vi "extracted json single string.vi"(7 "Data Type and Default Value":string, 9 "error in (no error)":errorcluster, 10 "Offset":i32, 11 "JSON":string) -> (1 "error out":errorcluster, 3 "Data out":string)   [LabVIEW 2026]
doc: "Convert JSON to the LabVIEW Data Type entered.\n\nStrings or Arrays of strings marked with a leading \"<JSON>\" tag in their name (including inside clusters) are returnd as JSON. \n\nStrings or Arrays of strings marked with a leading \"<UTF8>\" tag in their name (including inside clusters) are returned encoded as UTF-8 (rather than the standard LabVIEW encoding)."
uses:
  <vilib>/JDP Science/JSONtext/JSONtext.lvlib
  <vilib>/Utility/Data Type/NI_Data Type.lvlib
  <vilib>/JDP Science/JDP Science Common Utilities/JDP Utility.lvlib
  <vilib>/Utility/Data Type/Type Definitions/Data Type.ctl
  <vilib>/JDP Science/JSONtext/support/Tag Type.ctl
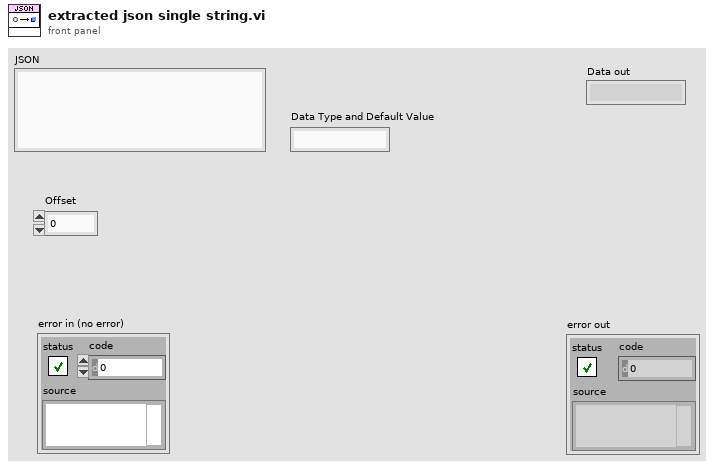
[diagram p1: front panel]
types:
  T1 = typedef "NI_Data Type.lvlib/Data Type.ctl" = enum8{"Invalid Type", "Void", "I8", "I16", "I32", "I64", "U8", "U16", "U32", "U64", "Single Float", "Double Float", "Extended Float", "Single Complex", "Double Complex", "Extended Complex", "Enum U8", "Enum U16", "Enum U32", "Enum U64", "Single Float With Unit", "Double Float With Unit", "Extended Float With Unit", "Single Complex with Unit", "Double Complex with Unit", "Extended Complex with Unit", "Boolean", "String", "Path", "Picture", "Tag", "Array", "Cluster", "Variant", "LV Variant", "Waveform", "Timestamp", "Digital Waveform", "Digital Data", "ExpressData", "Refnum", "External Data", "VI", "Poly VI", "LabVIEW Class Instance", "Fixed Point", "Set Collection", "Map Collection"}
  T2 = typedef "JSONtext.lvlib/Tag Type.ctl" = enum16{"No Tag", "<JSON>", "<JOBJ>", "<UTF8>"}
  T3 = enum16{"Parser Error", "Object", "Array", "String", "Number/Other", "Leading Whitespace", "Object end", "Array end", "Value end"}
  T4 = typedef "NI_Data Type.lvlib/Refnum Type.ctl" = enum16{"NotARefnum", "UnknownRefnum", "Generic", "Datalog", "ByteStream", "Device", "Occurence", "TCPNetConnection", "Auto", "Menu", "Imaq", "Hardware", "DataSocket", "Visa", "IVI", "UDPNetConnection", "Notifier", "Queue", "Irda", "EventReg", "DotNet", "UserEvent", "Callback", "UNUSED_EMPTY_POSITION", "BlueToothNetConnection", "LVObjApp", "LVObjVI", "LVObjUnknown", "GenericClass", "UserDefinedRefnumTag", "DataValue", "RT FIFO", "TDMS File", "PythonSessionRefnum"}
  T5 = typedef "JSONtext.lvlib/JSON Value Type.ctl" = enum16{"Not a JSON Value", "JSON Object", "JSON Array", "String", "Number", "true", "false", "null"}
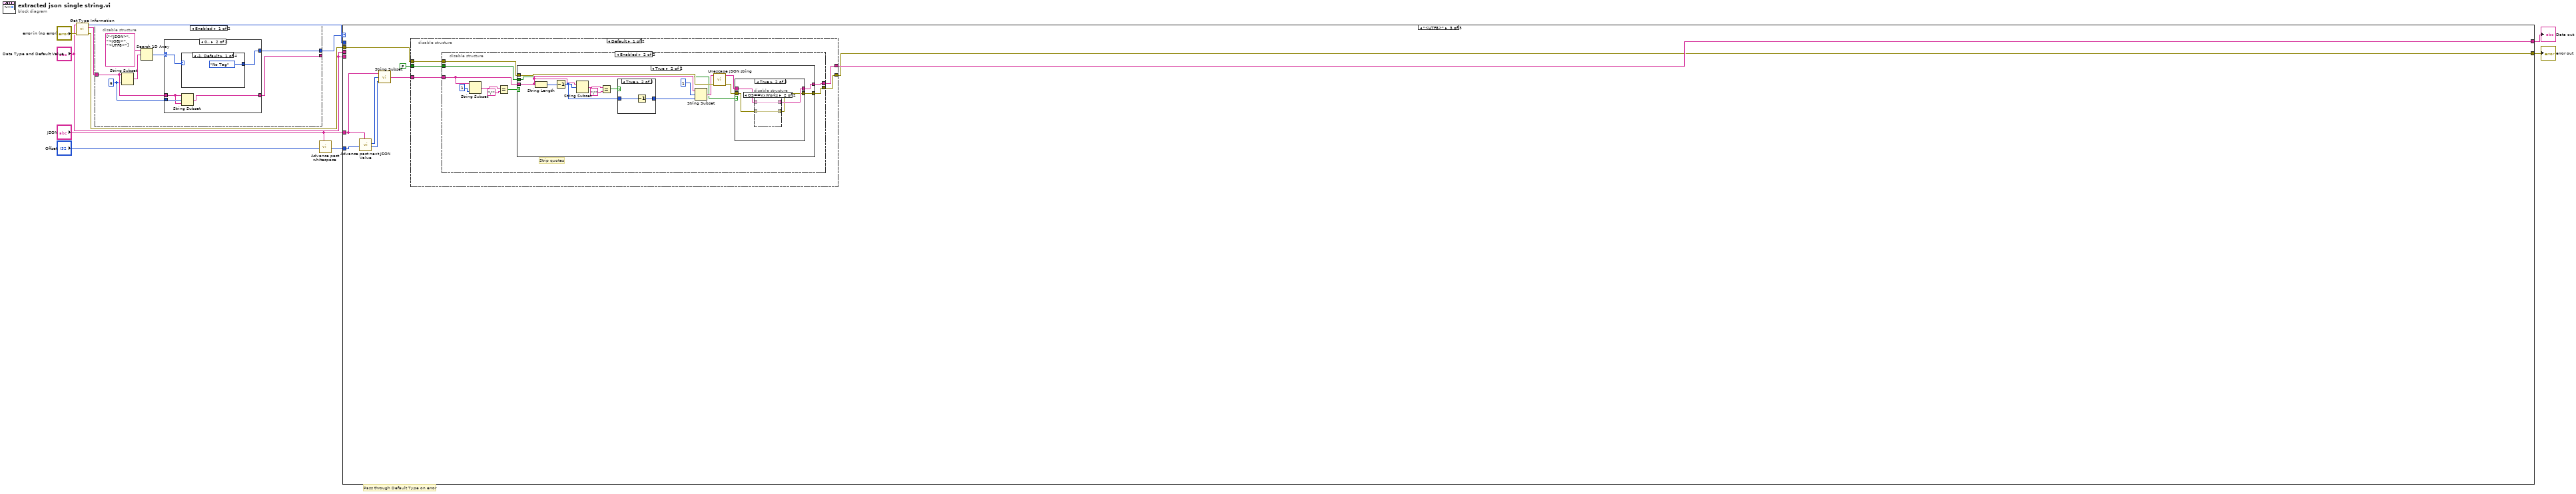
[diagram p0: block diagram]
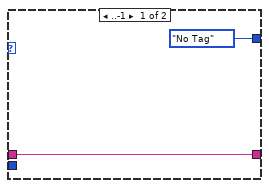
[diagram p2: hidden frame]
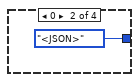
[diagram p3: hidden frame]
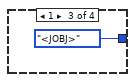
[diagram p4: hidden frame]
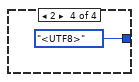
[diagram p5: hidden frame]
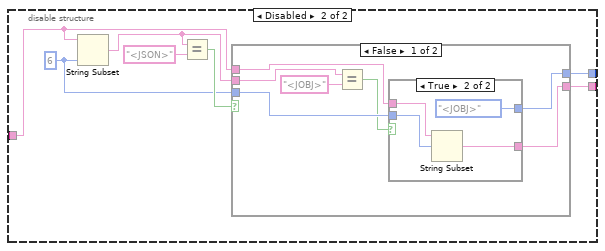
[diagram p6: hidden frame]
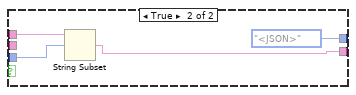
[diagram p8: hidden frame]
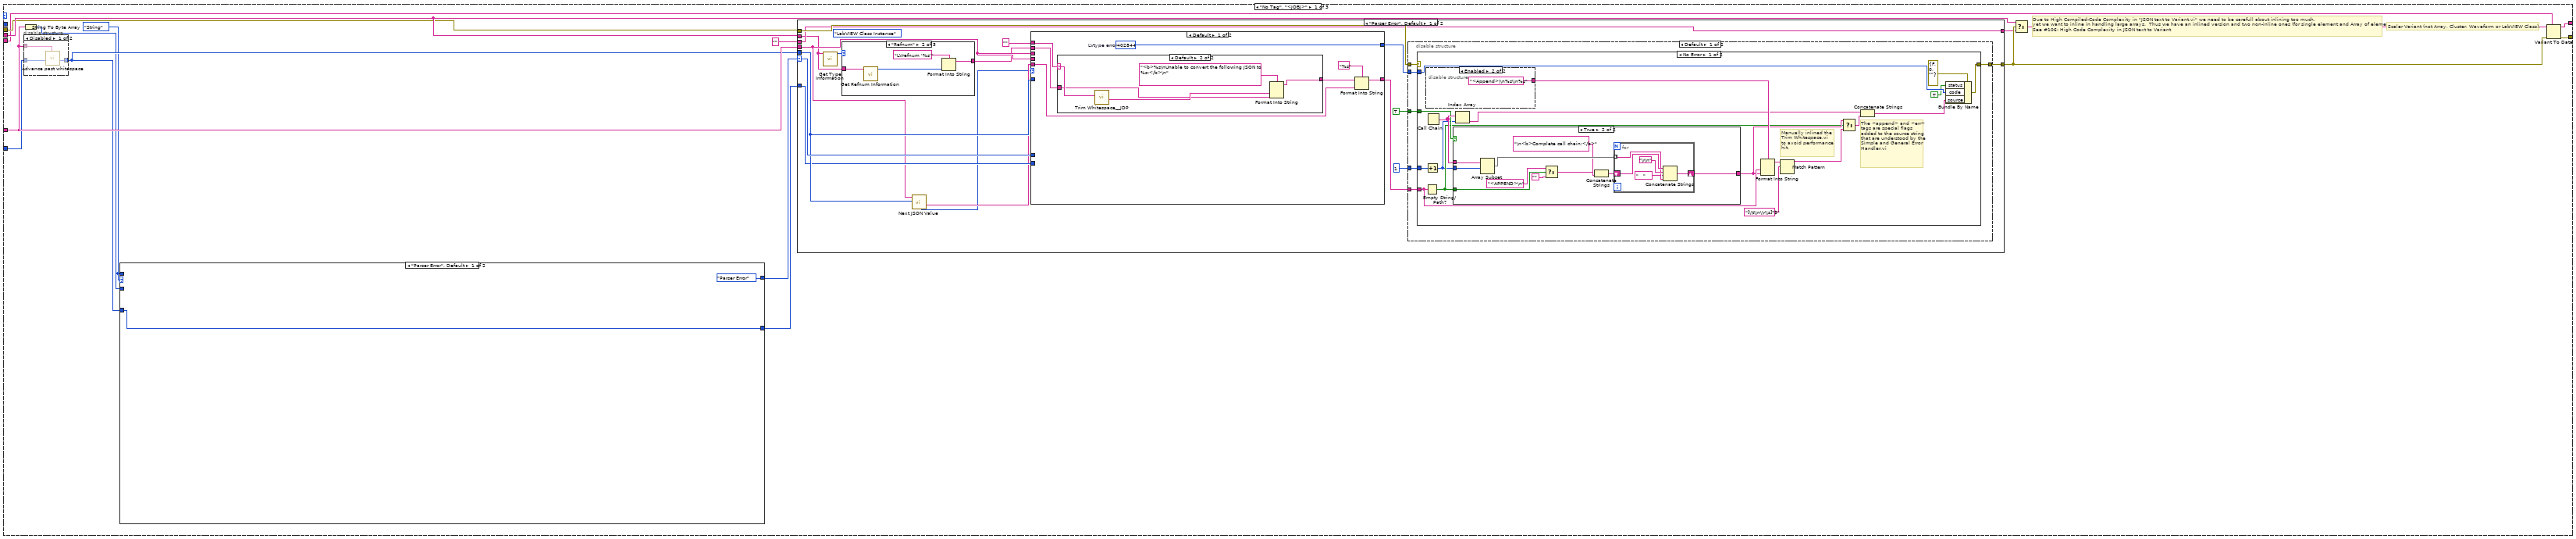
[diagram p9: hidden frame]
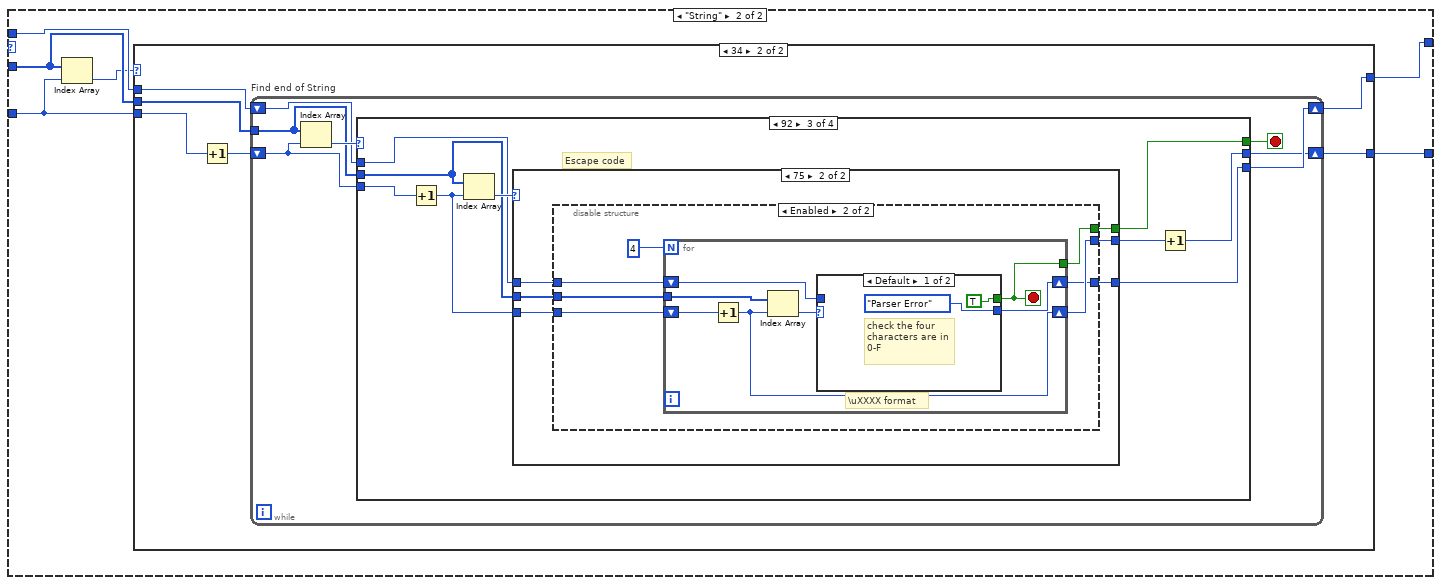
[diagram p10: hidden frame]
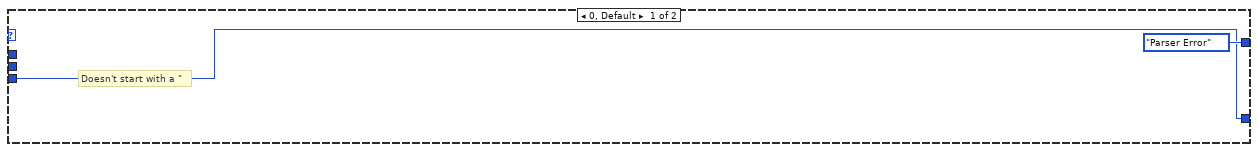
[diagram p11: hidden frame]
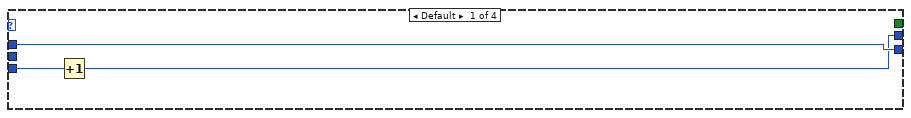
[diagram p12: hidden frame]
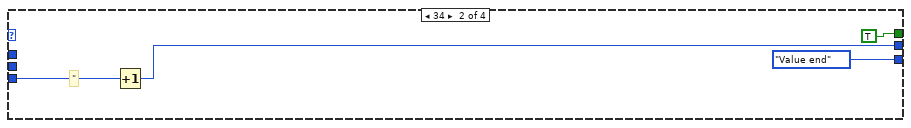
[diagram p13: hidden frame]
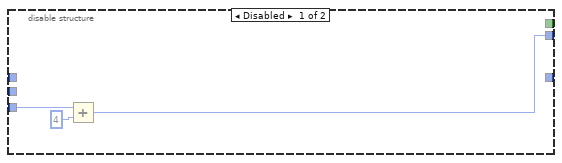
[diagram p15: hidden frame]
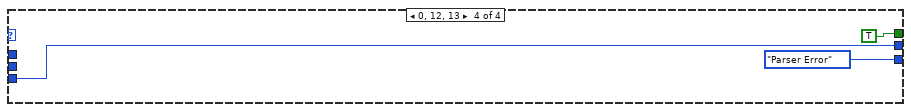
[diagram p17: hidden frame]
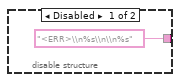
[diagram p18: hidden frame]
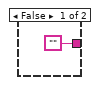
[diagram p19: hidden frame]
diagram:
  # "Pass through Default Type on error"
  n1 = call <vilib>:"Get Type Information.vi"("error in (no error)"="error in (no error)", "variant"="Data Type and Default Value") -> ("error out"=w4:errorcluster, "name"=w6:string, "type"=w3:T1)  [unwired: 5 in, 2 out]
  n2 = disable-structure shown="Enabled" {
    disable-tunnel: w6 -> [w18 w35]
    disable-tunnel: [w17 w34] -> _
    disable-tunnel: [w15 w30] -> w2
    frame Enabled {
      w16 = 6 ("length (rest)")
      n3 = String Subset(string=w18, length (rest)=w16) -> (substring=w13:string)  [unwired: 1 in]
      n4 = Search 1D Array(1D array=string[] ["<JSON>", "<JOBJ>", "<UTF8>"], element=w13) -> (index of element=w12:i32)  [unwired: 1 in]
      n5 = case shown="0.." w12 {
        selector: w12 -> [_ w23]
        tunnel: [w20 w25] -> w17
        tunnel: w18 -> [w20 w21]
        tunnel: w16 -> [_ w22]
        tunnel: [enum16{"No Tag", "<JSON>", "<JOBJ>", "<UTF8>"}."No Tag" ("Tag") w24] -> w15
        frame ..-1 {
        }
        frame 0.. {
          n6 = case shown="-1, Default" w23 {
            tunnel: [enum16{"No Tag", "<JSON>", "<JOBJ>", "<UTF8>"}."No Tag" ("Tag") enum16{"No Tag", "<JSON>", "<JOBJ>", "<UTF8>"}."<JSON>" ("Tag") enum16{"No Tag", "<JSON>", "<JOBJ>", "<UTF8>"}."<JOBJ>" ("Tag") enum16{"No Tag", "<JSON>", "<JOBJ>", "<UTF8>"}."<UTF8>" ("Tag")] -> w24
            frame -1, Default {
            }
            frame 0 {
            }
            frame 1 {
            }
            frame 2 {
            }
          }
          n7 = String Subset(string=w21, offset (0)=w22, length (rest)=w21) -> (substring=w25:string)
        }
      }
    }
    frame Disabled {
      w32 = 6 ("length (rest)")
      n8 = String Subset(string=w35, length (rest)=w32) -> (substring=w31:string)  [unwired: 1 in]
      n9 = Equal?(x=w31, y="<JSON>") -> (x = y?=w36:bool)
      n10 = case shown="False" w36 {
        tunnel: [w40 w51] -> w34
        tunnel: w35 -> [w41 w52]
        tunnel: w32 -> [w39 w50]
        tunnel: w31 -> [w42 _]
        tunnel: [w37 Tag_Type."<JSON>" ("Tag")] -> w30
        frame False {
          n11 = Equal?(x=w42, y="<JOBJ>") -> (x = y?=w38:bool)
          n12 = case shown="True" w38 {
            tunnel: w41 -> [w44 w48]
            tunnel: [w44 w47] -> w40
            tunnel: w39 -> [_ w46]
            tunnel: [_ Tag_Type."<JOBJ>" ("Tag")] -> w37
            frame False {
            }
            frame True {
              n13 = String Subset(string=w48, offset (0)=w46) -> (substring=w47:string)  [unwired: 1 in]
            }
          }
        }
        frame True {
          n14 = String Subset(string=w52, offset (0)=w50) -> (substring=w51:string)  [unwired: 1 in]
        }
      }
    }
  }
  n15 = call <vilib>:"Advance past whitespace.vi"("JSON"="JSON", "Offset"="Offset") -> ("Offset of first non-whitespace"=w5:i32)  [unwired: 7 in, 2 out]
  n16 = case shown="\"<UTF8>\"" w2 {
    tunnel: "Data Type and Default Value" -> [w68 _ _]
    tunnel: [w60 w376 w384] -> w8
    tunnel: "JSON" -> [w67 w377 w386]
    tunnel: w5 -> [w66 w380 w389]
    tunnel: w4 -> [w65 w375 w383]
    tunnel: [w63 w375 w382] -> w7
    tunnel: w3 -> [_ _ _]
    tunnel: "Data Type and Default Value" -> [w61 _ _]
    frame "No Tag", "<JOBJ>" {
      w54 = T3."String" ("State in")
      # "Scaler Variant (not Array, Cluster, Waveform or LabVIEW Class)."
      # "Due to High Compiled-Code Complexity in \"JSON text to Variant.vi\" we need to be carefull about inlining too much,\nyet we want to inline in handling large arrays.  Thus we have an inlined version and two non-inline ones (for single element and Array of elements)\nSee #106: High Code Complexity in JSON text to Variant"
      n17 = String To Byte Array(string=w67) -> (unsigned byte array=w53:u8[])
      n18 = disable-structure shown="Disabled" {
        disable-tunnel: w66 -> [w373 w374]
        disable-tunnel: [w372 w374] -> w59
        disable-tunnel: w67 -> [w371 _]
        frame Disabled {
          n19 = call <vilib>:"Advance past whitespace.vi"("JSON"=w371, "Offset"=w373) -> ("Offset of first non-whitespace"=w372:i32)  [unwired: 7 in, 2 out]
        }
        frame Enabled {
        }
      }
      n20 = case shown="\"Parser Error\", Default" w54 {
        tunnel: [T3."Parser Error" ("State in") w76] -> w55
        tunnel: [w70 w75] -> w56
        tunnel: w53 -> [_ w73]
        tunnel: w54 -> [_ w74]
        tunnel: w59 -> [w70 w72]
        frame "Parser Error", Default {
        }
        frame "String" {
          n21 = Index Array(array=w73, index=w72) -> (element=w71:u8)
          n22 = case shown="34" w71 {
            tunnel: [T3."Parser Error" ("State in") w84] -> w76
            tunnel: [w77 w83] -> w75
            tunnel: w74 -> [_ w82]
            tunnel: w73 -> [_ w80]
            tunnel: w72 -> [w77 w79]
            frame 0, Default {
              # "Doesn't start with a \""
            }
            frame 34 {
              n23 = Increment(x=w79) -> (x+1=w81:i32)
              n24 = while "Find end of String" {
                tunnel: w80 -> [w90]
                shift-right: [w85] -> w83
                shift-left: w81 -> [w86]
                shift-right: [w88] -> w84
                shift-left: w82 -> [w89]
                stop <- w87 stop-if-true
                n25 = Index Array(array=w90, index=w86) -> (element=w91:u8)
                n26 = case shown="92" w91 {
                  tunnel: w90 -> [_ _ w100 _]
                  tunnel: w89 -> [w94 _ w101 _]
                  tunnel: [w94 T3."Value end" w102 T3."Parser Error"] -> w88
                  tunnel: [_ TRUE w99 TRUE] -> w87
                  tunnel: w86 -> [w93 w96 w107 w138]
                  tunnel: [w92 w95 w103 w138] -> w85
                  frame Default {
                    n27 = Increment(x=w93) -> (x+1=w92:i32)
                  }
                  frame 34 {
                    # "\""
                    n28 = Increment(x=w96) -> (x+1=w95:i32)
                  }
                  frame 92 {
                    # "Escape code"
                    n29 = Increment(x=w107) -> (x+1=w105:i32)
                    n30 = Index Array(array=w100, index=w105) -> (element=w106:u8)
                    n31 = case shown="75" w106 {
                      tunnel: w105 -> [w109 w115]
                      tunnel: [w109 w114] -> w104
                      tunnel: [w108 w111] -> w102
                      tunnel: w101 -> [w108 w112]
                      tunnel: w100 -> [_ w113]
                      tunnel: [_ w110] -> w99
                      frame Default {
                        # "escaped character"
                      }
                      frame 117 {
                        n32 = disable-structure shown="Enabled" {
                          disable-tunnel: w115 -> [w118 w125]
                          disable-tunnel: [w116 w121] -> w114
                          disable-tunnel: w113 -> [_ w123]
                          disable-tunnel: w112 -> [_ w122]
                          disable-tunnel: [_ w120] -> w111
                          disable-tunnel: [_ w119] -> w110
                          frame Disabled {
                            n33 = Add(x=w118, y=4) -> (x+y=w116:i32)
                          }
                          frame Enabled {
                            n34 = for {
                              N: 4 -> [_]
                              tunnel: w123 -> [w130]
                              shift-right: [w128] -> w120
                              shift-left: w122 -> [w129]
                              shift-right: [w127] -> w121
                              shift-left: w125 -> [w132]
                              tunnel: [w126] -> w119
                              stop <- w126 stop-if-true
                              # "\\uXXXX format"
                              n35 = Increment(x=w132) -> (x+1=w127:i32)
                              n36 = Index Array(array=w130, index=w127) -> (element=w131:u8)
                              n37 = case shown="Default" w131 {
                                tunnel: w129 -> [_ w135]
                                tunnel: [T3."Parser Error" ("State in") w135] -> w128
                                tunnel: [TRUE _] -> w126
                                frame Default {
                                # "check the four\ncharacters are in\n0-F"
                                }
                                frame 48..57, 65..70, 97..102 {
                                # "0-9,A-F,a-f"
                                }
                              }
                            }
                          }
                        }
                      }
                    }
                    n38 = Increment(x=w104) -> (x+1=w103:i32)
                  }
                  frame 0, 12, 13 {
                  }
                }
              }
            }
          }
        }
      }
      n39 = case shown="\"Parser Error\", Default" w55 {
        selector: w55 -> [w153 _]
        tunnel: w67 -> [w150 w292]
        tunnel: [w155 w290] -> w64
        tunnel: w65 -> [w154 w291]
        tunnel: [w149 w289] -> w58
        tunnel: w59 -> [w152 w288]
        tunnel: w56 -> [w151 w287]
        tunnel: "" ("Data Type (default value)") -> [w149 _]
        tunnel: w68 -> [w148 _]
        frame "Parser Error", Default {
          (unwired) Data_Type."LabVIEW Class Instance" ("Type")
          n40 = call <vilib>:"Get Type Information.vi"("variant"=w148) -> ("type"=w143:T1)  [unwired: 6 in, 4 out]
          n41 = case shown="\"Refnum\"" w143 {
            selector: w143 -> [w274 _ _]
            tunnel: [w273 w277 w281] -> w146
            tunnel: w148 -> [_ w275 w285]
            frame Default {
              n42 = Format Into String(format string="LVType '%s'" ("initial string"), w274) -> (resulting string=w273:string)  [unwired: 2 in, 1 out]
            }
            frame "Refnum" {
              n43 = call <vilib>:"Get Refnum Information.vi"("variant"=w275) -> ("reference type"=w278:T4)  [unwired: 7 in, 3 out]
              n44 = Format Into String(format string="LVrefnum '%s'" ("initial string"), w278) -> (resulting string=w277:string)  [unwired: 2 in, 1 out]
            }
            frame "LabVIEW Class Instance" {
              n45 = Variant To Data(type=refnum<class> refnum ("LabVIEW Object"), Variant=w285) -> (data=w282:refnum<class>, error out=w283:errorcluster)  [unwired: 1 in]
              n46 = call <vilib>:"Get LV Class Name.vi"("error in (no error)"=w283, "object"=w282) -> ("class name"=w280:string)  [unwired: 8 in, 1 out]
              n47 = Format Into String(format string="Class '%s'" ("initial string"), w280) -> (resulting string=w281:string)  [unwired: 2 in, 1 out]
            }
          }
          n48 = call <vilib>:"Next JSON Value.vi"("Offset"=w152, "JSON"=w150) -> ("<JSON>"=w145:string, "JSON Value Type"=w144:T5)  [unwired: 6 in, 2 out]
          n49 = case shown="Default" w144 {
            tunnel: [w227 w261] -> w139
            tunnel: w150 -> [_ w260]
            tunnel: w151 -> [_ w259]
            tunnel: [w226 w258] -> w142
            tunnel: w150 -> [_ _]
            tunnel: w152 -> [_ w242]
            tunnel: w145 -> [w228 _]
            tunnel: "" ("initial string") -> [w223 w238]
            tunnel: w153 -> [_ w241]
            tunnel: w146 -> [w224 w239]
            frame Default {
              w226 = 402844  # LVtype error
              n50 = case shown="Default" w223 {
                selector: w223 -> [_ w237]
                tunnel: [w230 w236] -> w225
                tunnel: w224 -> [w232 w233]
                frame "" {
                  n51 = Format Into String(format string="<b>Unable to convert the following JSON to %s:</b>\n", w232) -> (resulting string=w230:string)  [unwired: 2 in, 1 out]
                }
                frame Default {
                  n52 = call <vilib>:"Trim Whitespace__JDP.vi"("String in"=w237) -> ("String out"=w234:string)  [unwired: 6 in]
                  n53 = Format Into String(format string="<b>%s\nUnable to convert the following JSON to %s:</b>\n", w234, w233) -> (resulting string=w236:string)  [unwired: 2 in, 1 out]
                }
              }
              n54 = Format Into String(format string="%s", initial string=w225, w228) -> (resulting string=w227:string)  [unwired: 1 in, 1 out]
            }
            frame "Not a JSON Value" {
              w258 = 402841  # Parsing Error
              n55 = case shown="Default" w238 {
                selector: w238 -> [_ w269]
                tunnel: [w262 w268] -> w240
                tunnel: w239 -> [w264 w265]
                frame "" {
                  n56 = Format Into String(format string="<b>Error converting to %s:</b>\n", w264) -> (resulting string=w262:string)  [unwired: 2 in, 1 out]
                }
                frame Default {
                  n57 = call <vilib>:"Trim Whitespace__JDP.vi"("String in"=w269) -> ("String out"=w266:string)  [unwired: 6 in]
                  n58 = Format Into String(format string="<b>%s</b>\nError converting to %s:\n", w266, w265) -> (resulting string=w268:string)  [unwired: 2 in, 1 out]
                }
              }
              n59 = String Length(string=w260) -> (length=w243:i32)
              n60 = Subtract(x=w259, y=100) -> (x-y=w255:i32)
              n61 = case shown="Default" w243 {
                tunnel: ["Parser State: '%s', near <b>¿¿¿</b> marker in:\n<b>'%s¿¿¿</b>%s'\n" ("format string") "Parser State: '%s', in:\n<b>'%s</b>%s'\n" ("format string")] -> w244
                frame 20.. {
                }
                frame Default {
                }
              }
              n62 = Max & Min(x=w255, y=w242) -> (max(x,y)=w246:i32)  [unwired: 1 out]
              n63 = Subtract(x=w259, y=30) -> (x-y=w247:i32)
              n64 = Max & Min(x=w246, y=w247) -> (max(x,y)=w245:i32)  [unwired: 1 out]
              n65 = Max & Min(x=w245, y=0) -> (max(x,y)=w253:i32)  [unwired: 1 out]
              n66 = call <vilib>:"String Subset.vi"("Offset past End"=w259, "Start offset"=w253, "JSON"=w260) -> ("substring"=w251:string)  [unwired: 2 in]
              n67 = String Length(string=w251) -> (length=w252:i32)
              n68 = Add(x=w253, y=w252) -> (x+y=w250:i32)
              n69 = String Subset(string=w260, offset (0)=w250, length (rest)=30 ("Offset past End")) -> (substring=w257:string)
              n70 = Format Into String(format string=w244, initial string=w240, w241, w251, w257) -> (resulting string=w261:string)  [unwired: 1 in, 1 out]
            }
          }
          n71 = disable-structure shown="Default" {
            disable-tunnel: [w161 w201] -> w155
            disable-tunnel: w154 -> [w160 w202]
            disable-tunnel: w142 -> [w159 w200]
            disable-tunnel: w139 -> [w158 _]
            disable-tunnel: 1 ("Call Depth") -> [w157 _]
            disable-tunnel: TRUE ("show call chain? (False)") -> [w156 _]
            frame condition #0 (active) {
              n72 = case shown="No Error" w160 {
                selector: w160 -> [_ w198]
                tunnel: [w179 w198] -> w161
                tunnel: w159 -> [w178 _]
                tunnel: w158 -> [w177 _]
                tunnel: w157 -> [w176 _]
                tunnel: w156 -> [w172 _]
                frame No Error {
                  # "Manually inlined the\nTrim Whitespace.vi\nto avoid performance\nhit."
                  # "The <append> and <err> tags are special flags added to the source string that are understood by the Simple and General Error Handler.vi"
                  n73 = Empty String/Path?(string/path=w177) -> (empty?=w168:bool)
                  n74 = Increment(x=w176) -> (x+1=w163:i32)
                  n75 = disable-structure shown="Enabled" {
                    disable-tunnel: ["<ERR>\\n%s\\n\\n%s" ("format string") "<Append>\\n%s\\n%s" ("format string")] -> w171
                    frame Disabled {
                    }
                    frame Enabled {
                    }
                  }
                  n76 = Call Chain() -> (call chain=w173:string[])
                  n77 = case shown="True" w172 {
                    tunnel: ["" w192] -> w170
                    tunnel: w173 -> [_ w191]
                    tunnel: w168 -> [_ w187]
                    tunnel: w163 -> [_ w183]
                    frame False {
                    }
                    frame True {
                      n78 = Array Subset(array=w191, index=w183) -> (w190:string[])  [unwired: 1 in]
                      n79 = Select(t="<APPEND>\n", s=w187, f="") -> (s? t:f=w184:string)
                      n80 = Concatenate Strings(w184, "\n<b>Complete call chain:</b>" ("call chain header")) -> (w188:string)
                      n81 = for {
                        tunnel: w190 -> [w194] mode=indexing
                        shift-right: [w197] -> w192
                        shift-left: w188 -> [w195]
                        n82 = Concatenate Strings(w195, "\r\n", "   ", w194) -> (w197:string)
                      }
                    }
                  }
                  n83 = Index Array(array=w173, index=w163) -> (element=w164:string)
                  n84 = Format Into String(format string=w171, w177, w170) -> (resulting string=w166:string)  [unwired: 2 in, 1 out]
                  n85 = Match Pattern(string=w166, regular expression="[\\t\\n\\r\\s]*$") -> (before substring=w165:string)  [unwired: 1 in, 3 out]
                  n86 = Select(t=w170, s=w168, f=w165) -> (s? t:f=w169:string)
                  n87 = Concatenate Strings(w164, w169) -> (w174:string)
                  n88 = Bundle By Name(cluster=errorcluster {"status"=FALSE, "code"=0, "source"=""} ("error out"), "status"=TRUE, "code"=w178, "source"=w174) -> (w179:errorcluster)
                }
                frame Error {
                  # "An error in trumps any error code input."
                }
              }
            }
            frame condition #1 {
              n89 = case shown="Default" w200 {
                selector: w200 -> [_ w205]
                tunnel: w202 -> [w203 w207]
                tunnel: [w203 w206] -> w201
                tunnel: [_ w204] -> w199
                frame 0 {
                  # "If the error code in equals zero, then propagate the error in cluster regardless of its value."
                }
                frame Default {
                  n90 = case shown="No Error" w207 {
                    selector: w207 -> [w209 w222]
                    tunnel: [w213 w222] -> w206
                    tunnel: w205 -> [w214 _]
                    tunnel: w204 -> [w210 _]
                    frame No Error {
                      n91 = Unbundle By Name(w209) -> ("code"=w212:i32)
                      n92 = Not Equal To 0?(x=w212) -> (x != 0?=w211:bool)
                      n93 = And(x=w210, y=w211) -> (x .and. y?=w208:bool)
                      n94 = case shown="False" w208 {
                        tunnel: w214 -> [w220 _]
                        tunnel: [w217 w221] -> w213
                        tunnel: w210 -> [w216 _]
                        tunnel: w209 -> [w215 w221]
                        frame False {
                          n95 = Not(x=w216) -> (.not. x?=w219:bool)
                          n96 = Bundle By Name(cluster=w215, "status"=w219, "code"=w220, "source"="Error Cluster From Error Code.vi") -> (w217:errorcluster)
                        }
                        frame True {
                          # "If the error code input is setting a warning, and a warning is already set on the wire, then we\ngo with the one already on the wire."
                        }
                      }
                    }
                    frame Error {
                      # "An error in trumps any error code input."
                    }
                  }
                }
              }
            }
          }
        }
        frame "Value end" {
          n97 = call <vilib>:"String Subset.vi"("Offset past End"=w287, "Start offset"=w288, "JSON"=w292) -> ("substring"=w293:string)  [unwired: 2 in]
          n98 = disable-structure shown="Default" {
            disable-tunnel: [w298 w366] -> w290
            disable-tunnel: w291 -> [w297 w368]
            disable-tunnel: [w296 w367] -> w289
            disable-tunnel: w293 -> [w295 w370]
            disable-tunnel: TRUE ("To System Encoding (T)") -> [w294 _]
            frame condition #0 (active) {
              n99 = disable-structure shown="Enabled" {
                disable-tunnel: [w307 w333] -> w298
                disable-tunnel: w297 -> [w305 w332]
                disable-tunnel: [w304 w331] -> w296
                disable-tunnel: w295 -> [w299 w329]
                disable-tunnel: w294 -> [_ w325]
                frame Disabled {
                  # "Strip quotes"
                  n100 = Search and Replace String(input string=w299, search string="^\"", error in=w305) -> (result string=w303:string, number of replacements=w301:i32, error out=w306:errorcluster)  [unwired: 5 in, 1 out]
                  n101 = Greater Than 0?(x=w301) -> (x > 0?=w300:bool)
                  n102 = case shown="True" w300 {
                    tunnel: [w308 w310] -> w307
                    tunnel: w306 -> [w308 w318]
                    tunnel: [w309 w312] -> w304
                    tunnel: w303 -> [w309 w317]
                    frame False {
                      # "Not a leading quote?   This shouldn't happen."
                    }
                    frame True {
                      n103 = Search and Replace String(input string=w317, search string="\"$", error in=w318) -> (result string=w315:string, error out=w314:errorcluster)  [unwired: 5 in, 2 out]
                      n104 = call <vilib>:"Unescape JSON string.vi"("error in (no error)"=w314, "Text (with JSON escapes)"=w315) -> ("error out"=w311:errorcluster, "Text (unescaped)"=w313:string)  [unwired: 8 in]
                      n105 = disable-structure shown="Default" {
                        disable-tunnel: w313 -> [w322 w324]
                        disable-tunnel: [w321 w324] -> w312
                        disable-tunnel: w311 -> [w320 w323]
                        disable-tunnel: [w319 w323] -> w310
                        frame condition #0 (active) {
                          n106 = UTF-8 to Text(8:w320, 11:w322) -> (0:w319:errorcluster, 3:w321:string)  [unwired: 1 in]
                        }
                        frame condition #1 {
                        }
                      }
                    }
                  }
                }
                frame Enabled {
                  # "Strip quotes"
                  n107 = String Subset(string=w329, length (rest)=1 ("length (rest)")) -> (substring=w328:string)  [unwired: 1 in]
                  n108 = Equal?(x=w328, y="\"") -> (x = y?=w326:bool)
                  n109 = case shown="True" w326 {
                    tunnel: [w334 w346] -> w333
                    tunnel: w332 -> [w334 w350]
                    tunnel: [w335 w348] -> w331
                    tunnel: w329 -> [w335 w342]
                    tunnel: w325 -> [_ w336]
                    frame False {
                    }
                    frame True {
                      n110 = String Length(string=w342) -> (length=w343:i32)
                      n111 = Decrement(x=w343) -> (x-1=w339:i32)
                      n112 = String Subset(string=w342, offset (0)=w339) -> (substring=w344:string)  [unwired: 1 in]
                      n113 = Equal?(x=w344, y="\"") -> (x = y?=w337:bool)
                      n114 = case shown="True" w337 {
                        tunnel: w339 -> [w363 w365]
                        tunnel: [w363 w364] -> w338
                        frame False {
                        }
                        frame True {
                          n115 = Decrement(x=w365) -> (x-1=w364:i32)
                        }
                      }
                      n116 = String Subset(string=w342, offset (0)=1, length (rest)=w338) -> (substring=w340:string)
                      n117 = call <vilib>:"Unescape JSON string.vi"("error in (no error)"=w350, "Text (with JSON escapes)"=w340) -> ("error out"=w347:errorcluster, "Text (unescaped)"=w349:string)  [unwired: 8 in]
                      n118 = case shown="True" w336 {
                        tunnel: w349 -> [w352 w356]
                        tunnel: [w352 w355] -> w348
                        tunnel: w347 -> [w351 w354]
                        tunnel: [w351 w353] -> w346
                        frame False {
                        }
                        frame True {
                          n119 = disable-structure shown="OS==VxWorks" {
                            disable-tunnel: w356 -> [w360 w362]
                            disable-tunnel: [w359 w362] -> w355
                            disable-tunnel: w354 -> [w358 w361]
                            disable-tunnel: [w357 w361] -> w353
                            frame condition #0 (active) {
                              n120 = UTF-8 to Text(8:w358, 11:w360) -> (0:w357:errorcluster, 3:w359:string)  [unwired: 1 in]
                            }
                            frame condition #1 {
                            }
                          }
                        }
                      }
                    }
                  }
                }
              }
            }
            frame condition #1 {
              # "Stopgap, since VxWorks does not support UTF8 function:\n\nWarning: inherits the \\u0000 bug"
              n121 = Unflatten From JSON(JSON string=w370, type and defaults="", error in (no error)=w368) -> (value=w367:string, error out=w366:errorcluster)  [unwired: 4 in]
            }
          }
        }
      }
      n122 = Select(t=w68, s=w64, f=w58) -> (s? t:f=w62:string)
      n123 = Variant To Data(error in=w64, type=w61, Variant=w62) -> (data=w60:string, error out=w63:errorcluster)
    }
    frame "<JSON>" {
      n124 = call <vilib>:"Advance past next JSON Value.vi"("JSON"=w377, "Offset"=w380) -> ("Offset out"=w379:i32, "Value start"=w378:i32)  [unwired: 7 in, 1 out]
      n125 = call <vilib>:"String Subset.vi"("Offset past End"=w379, "Start offset"=w378, "JSON"=w377) -> ("substring"=w376:string)  [unwired: 2 in]
    }
    frame "<UTF8>" {
      n126 = call <vilib>:"Advance past next JSON Value.vi"("JSON"=w386, "Offset"=w389) -> ("Offset out"=w388:i32, "Value start"=w387:i32)  [unwired: 7 in, 1 out]
      n127 = call <vilib>:"String Subset.vi"("Offset past End"=w388, "Start offset"=w387, "JSON"=w386) -> ("substring"=w385:string)  [unwired: 2 in]
      n128 = disable-structure shown="Default" {
        disable-tunnel: [w394 w462] -> w382
        disable-tunnel: w383 -> [w393 w464]
        disable-tunnel: [w392 w463] -> w384
        disable-tunnel: w385 -> [w391 w466]
        disable-tunnel: FALSE ("To System Encoding (T)") -> [w390 _]
        frame condition #0 (active) {
          n129 = disable-structure shown="Enabled" {
            disable-tunnel: [w403 w429] -> w394
            disable-tunnel: w393 -> [w401 w428]
            disable-tunnel: [w400 w427] -> w392
            disable-tunnel: w391 -> [w395 w425]
            disable-tunnel: w390 -> [_ w421]
            frame Disabled {
              # "Strip quotes"
              n130 = Search and Replace String(input string=w395, search string="^\"", error in=w401) -> (result string=w399:string, number of replacements=w397:i32, error out=w402:errorcluster)  [unwired: 5 in, 1 out]
              n131 = Greater Than 0?(x=w397) -> (x > 0?=w396:bool)
              n132 = case shown="True" w396 {
                tunnel: [w404 w406] -> w403
                tunnel: w402 -> [w404 w414]
                tunnel: [w405 w408] -> w400
                tunnel: w399 -> [w405 w413]
                frame False {
                  # "Not a leading quote?   This shouldn't happen."
                }
                frame True {
                  n133 = Search and Replace String(input string=w413, search string="\"$", error in=w414) -> (result string=w411:string, error out=w410:errorcluster)  [unwired: 5 in, 2 out]
                  n134 = call <vilib>:"Unescape JSON string.vi"("error in (no error)"=w410, "Text (with JSON escapes)"=w411) -> ("error out"=w407:errorcluster, "Text (unescaped)"=w409:string)  [unwired: 8 in]
                  n135 = disable-structure shown="Default" {
                    disable-tunnel: w409 -> [w418 w420]
                    disable-tunnel: [w417 w420] -> w408
                    disable-tunnel: w407 -> [w416 w419]
                    disable-tunnel: [w415 w419] -> w406
                    frame condition #0 (active) {
                      n136 = UTF-8 to Text(8:w416, 11:w418) -> (0:w415:errorcluster, 3:w417:string)  [unwired: 1 in]
                    }
                    frame condition #1 {
                    }
                  }
                }
              }
            }
            frame Enabled {
              # "Strip quotes"
              n137 = String Subset(string=w425, length (rest)=1 ("length (rest)")) -> (substring=w424:string)  [unwired: 1 in]
              n138 = Equal?(x=w424, y="\"") -> (x = y?=w422:bool)
              n139 = case shown="True" w422 {
                tunnel: [w430 w442] -> w429
                tunnel: w428 -> [w430 w446]
                tunnel: [w431 w444] -> w427
                tunnel: w425 -> [w431 w438]
                tunnel: w421 -> [_ w432]
                frame False {
                }
                frame True {
                  n140 = String Length(string=w438) -> (length=w439:i32)
                  n141 = Decrement(x=w439) -> (x-1=w435:i32)
                  n142 = String Subset(string=w438, offset (0)=w435) -> (substring=w440:string)  [unwired: 1 in]
                  n143 = Equal?(x=w440, y="\"") -> (x = y?=w433:bool)
                  n144 = case shown="True" w433 {
                    tunnel: w435 -> [w459 w461]
                    tunnel: [w459 w460] -> w434
                    frame False {
                    }
                    frame True {
                      n145 = Decrement(x=w461) -> (x-1=w460:i32)
                    }
                  }
                  n146 = String Subset(string=w438, offset (0)=1, length (rest)=w434) -> (substring=w436:string)
                  n147 = call <vilib>:"Unescape JSON string.vi"("error in (no error)"=w446, "Text (with JSON escapes)"=w436) -> ("error out"=w443:errorcluster, "Text (unescaped)"=w445:string)  [unwired: 8 in]
                  n148 = case shown="True" w432 {
                    tunnel: w445 -> [w448 w452]
                    tunnel: [w448 w451] -> w444
                    tunnel: w443 -> [w447 w450]
                    tunnel: [w447 w449] -> w442
                    frame False {
                    }
                    frame True {
                      n149 = disable-structure shown="OS==VxWorks" {
                        disable-tunnel: w452 -> [w456 w458]
                        disable-tunnel: [w455 w458] -> w451
                        disable-tunnel: w450 -> [w454 w457]
                        disable-tunnel: [w453 w457] -> w449
                        frame condition #0 (active) {
                          n150 = UTF-8 to Text(8:w454, 11:w456) -> (0:w453:errorcluster, 3:w455:string)  [unwired: 1 in]
                        }
                        frame condition #1 {
                        }
                      }
                    }
                  }
                }
              }
            }
          }
        }
        frame condition #1 {
          # "Stopgap, since VxWorks does not support UTF8 function:\n\nWarning: inherits the \\u0000 bug"
          n151 = Unflatten From JSON(JSON string=w466, type and defaults="", error in (no error)=w464) -> (value=w463:string, error out=w462:errorcluster)  [unwired: 4 in]
        }
      }
    }
  }
  "Data out" <- w8
  "error out" <- w7
